vi "DGHD5331_timestamp.vi"() -> ()   [LabVIEW 2014]
uses:
  <vilib>/Instr/_visa.llb/VISA Configure Serial Port (Instr).vi
  <vilib>/Utility/file.llb/Write To Spreadsheet File (string).vi
panel:
  out "No of samples":i32
  out "Time/Date":string
  out "Raw Data Read":string
  out "Run time (sec)":dbl
  out "Bytes Read":u32
  in  "Comm Port":refnum<visa-resource-name>
  in  "Sample rate (s)":u8=232 min=255 step=255
  out "Waveform Chart":dynamicdata(graph)
  in  "stop":bool
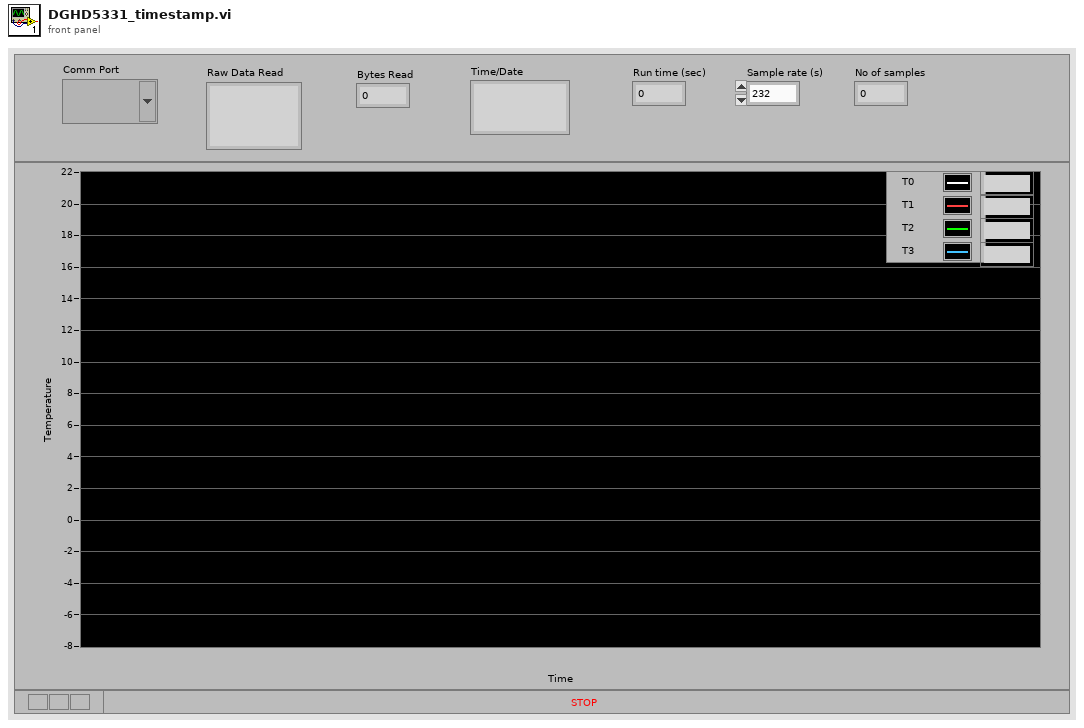
[diagram p1: front panel]
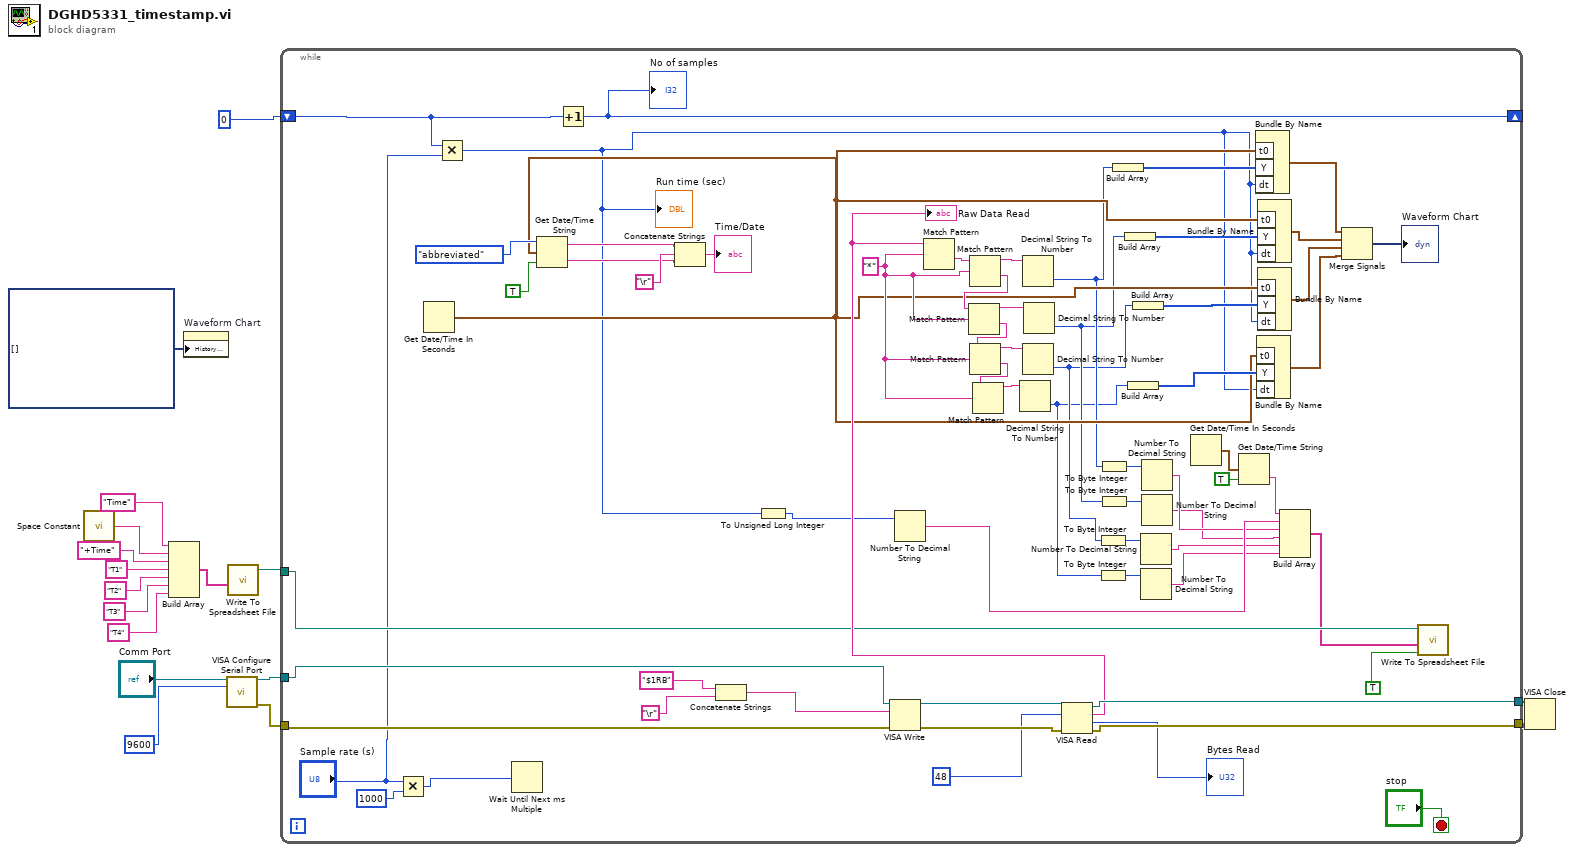
[diagram p0: block diagram]
diagram:
  n1 = call <vilib>:"Space Constant.vi"() -> ("String"=w2:string)
  n2 = Build Array("Time" ("element"), w2, "+Time", "T1", "T2", "T3", "T4") -> (w6:string[])
  n3 = property on="Waveform Chart" class="WFChart (strict)"("History Data"=dynamicdata[] []) -> ()  [unwired: 2 in, 2 out]
  n4 = call-poly "VISA Configure Serial Port"("VISA resource name"="Comm Port", "baud rate (9600)"=9600) -> ("VISA resource name out"=w16:refnum<visa-resource-name>, "error out"=w14:errorcluster)  [unwired: 12 in]
  n5 = call-poly <vilib>:"Write To Spreadsheet File.vi"("1D data"=w6) -> ("new file path (Not A Path if cancelled)"=w4:path)  [unwired: 7 in]
  n6 = while {
    tunnel: w16 -> [w80]
    tunnel: w14 -> [w79]
    tunnel: [w76] -> w13
    tunnel: [w75] -> w12
    shift-right: [w60] -> _
    shift-left: 0 -> [w43]
    tunnel: w4 -> [w42]
    stop <- "stop" stop-if-true
    w64 = "*"
    n7 = Multiply(x="Sample rate (s)", y=1000) -> (x*y=w20:i32)
    n8 = Get Date/Time In Seconds() -> (seconds since 1Jan1904=w47:timestamp)
    n9 = Multiply(x=w43, y="Sample rate (s)") -> (x*y=w18:i32)
    "Run time (sec)" <- w18
    n10 = Wait Until Next ms Multiple(millisecond multiple=w20) -> ()  [unwired: 1 out]
    n11 = Get Date/Time String(date format (0)=enum16{"short", "long", "abbreviated"}."abbreviated", seconds (now)=w47, want seconds? (F)=TRUE) -> (date string=w41:string, time string=w40:string)
    n12 = Increment(x=w43) -> (x+1=w60:i32)
    "No of samples" <- w60
    n13 = Concatenate Strings(w41, "\r", w40) -> (→"Time/Date":string)
    n14 = Concatenate Strings("$1RB", "\r") -> (w71:string)
    n15 = To Unsigned Long Integer(number=w18) -> (unsigned 32bit integer=w36:u32)
    n16 = VISA Write(VISA resource name=w80, write buffer=w71, error in (no error)=w79) -> (VISA resource name out=w78:refnum<visa-resource-name>, error out=w77:errorcluster)  [unwired: 1 out]
    n17 = Number To Decimal String(number=w36) -> (decimal integer string=w35:string)  [unwired: 1 in]
    n18 = VISA Read(VISA resource name=w78, byte count=u32 48 ("Bytes Read"), error in (no error)=w77) -> (VISA resource name out=w76:refnum<visa-resource-name>, read buffer=w59:string, return count=→"Bytes Read":u32, error out=w75:errorcluster)
    "Raw Data Read" <- w59
    n19 = Match Pattern(string=w59, regular expression=w64) -> (after substring=w70:string)  [unwired: 1 in, 3 out]
    n20 = Match Pattern(string=w70, regular expression=w64) -> (before substring=w69:string, after substring=w67:string)  [unwired: 1 in, 2 out]
    n21 = Match Pattern(string=w67, regular expression=w64) -> (before substring=w68:string, after substring=w63:string)  [unwired: 1 in, 2 out]
    n22 = Match Pattern(string=w63, regular expression=w64) -> (before substring=w66:string, after substring=w62:string)  [unwired: 1 in, 2 out]
    n23 = Match Pattern(string=w62, regular expression=w64) -> (before substring=w65:string)  [unwired: 1 in, 3 out]
    n24 = Decimal String To Number(string=w65) -> (number=w27:i32)  [unwired: 2 in, 1 out]
    n25 = Decimal String To Number(string=w69) -> (number=w30:i32)  [unwired: 2 in, 1 out]
    n26 = Decimal String To Number(string=w66) -> (number=w28:i32)  [unwired: 2 in, 1 out]
    n27 = Decimal String To Number(string=w68) -> (number=w29:i32)  [unwired: 2 in, 1 out]
    n28 = To Byte Integer(number=w28) -> (8bit integer=w32:i8)
    n29 = To Byte Integer(number=w27) -> (8bit integer=w31:i8)
    n30 = To Byte Integer(number=w30) -> (8bit integer=w34:i8)
    n31 = To Byte Integer(number=w29) -> (8bit integer=w33:i8)
    n32 = Build Array(w30) -> (w55:i32[])
    n33 = Build Array(w29) -> (w54:i32[])
    n34 = Build Array(w27) -> (w52:i32[])
    n35 = Build Array(w28) -> (w53:i32[])
    n36 = Number To Decimal String(number=w32) -> (decimal integer string=w24:string)  [unwired: 1 in]
    n37 = Number To Decimal String(number=w31) -> (decimal integer string=w23:string)  [unwired: 1 in]
    n38 = Number To Decimal String(number=w34) -> (decimal integer string=w26:string)  [unwired: 1 in]
    n39 = Number To Decimal String(number=w33) -> (decimal integer string=w25:string)  [unwired: 1 in]
    n40 = Get Date/Time In Seconds() -> (seconds since 1Jan1904=w38:timestamp)
    n41 = Get Date/Time String(seconds (now)=w38, want seconds? (F)=TRUE) -> (time string=w37:string)  [unwired: 1 in, 1 out]
    n42 = Bundle By Name("t0"=w47, "Y"=w55, "dt"=w18) -> (w46:waveform(i32))  [unwired: 1 in]
    n43 = Bundle By Name("t0"=w47, "Y"=w52, "dt"=w18) -> (w48:waveform(i32))  [unwired: 1 in]
    n44 = Bundle By Name("t0"=w47, "Y"=w54, "dt"=w18) -> (w45:waveform(i32))  [unwired: 1 in]
    n45 = Bundle By Name("t0"=w47, "Y"=w53, "dt"=w18) -> (w44:waveform(i32))  [unwired: 1 in]
    n46 = Build Array(w37, w35, w26, w25, w24, w23) -> (w39:string[])
    n47 = Merge Signals(w46, w45, w44, w48) -> (→"Waveform Chart":dynamicdata)
    n48 = call-poly <vilib>:"Write To Spreadsheet File.vi"("append to file? (new file:F)"=TRUE, "1D data"=w39, "file path (dialog if empty)"=w42) -> ()  [unwired: 5 in, 1 out]
  }
  n49 = VISA Close(VISA resource name=w13, error in (no error)=w12) -> ()  [unwired: 1 out]
